vi "Update.vi"() -> ()   [LabVIEW 2015]
uses:
  <vilib>/zip/NI_Unzip.lvlib
panel:
  out "String":string
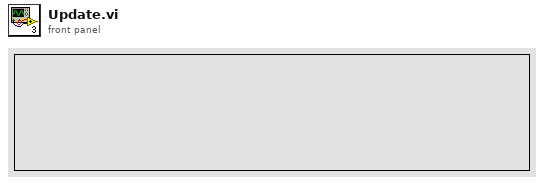
[diagram p1: front panel]
types:
  T1 = enum16{"open", "replace", "create", "open or create", "replace or create", "replace or create with confirmation"}
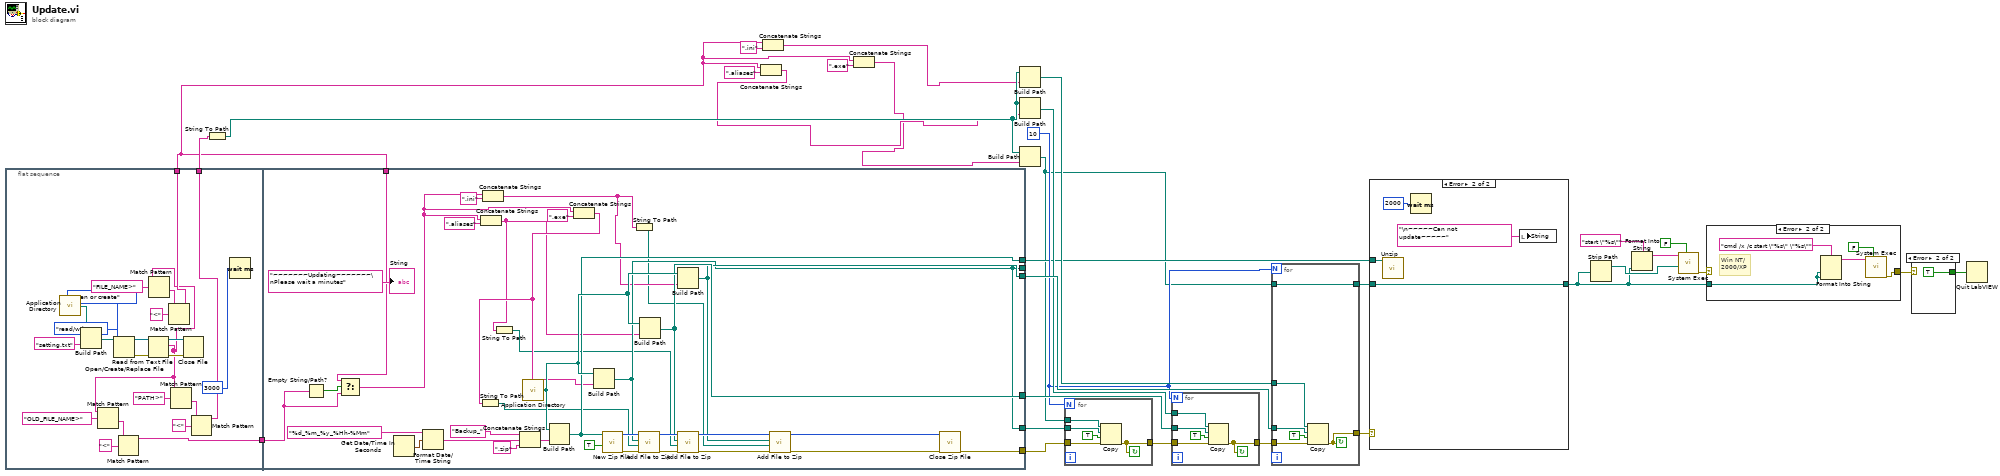
[diagram p0: block diagram]
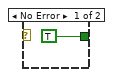
[diagram p2: hidden frame]
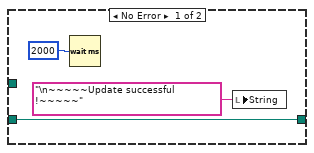
[diagram p4: hidden frame]
diagram:
  w23 = 10
  n1 = flat-sequence {
    tunnel: [w41] -> w7
    tunnel: [w37] -> w2
    tunnel: [w32] -> w3
    tunnel: [w68] -> w31
    tunnel: [w74] -> w30
    tunnel: [w73] -> w29
    tunnel: [w71] -> w28
    tunnel: [w70] -> w22
    tunnel: [w68] -> _
    tunnel: w3 -> [w65]
    tunnel: w2 -> [w66]
    frame #0 {
      n2 = call <vilib>:"Application Directory.vi"() -> ("Application Directory"=w53:path)
      n3 = Build Path(base path=w53, name or relative path="setting.txt") -> (appended path=w51:path)
      n4 = Open/Create/Replace File(file path (use dialog)=w51, operation (0:open)=T1."open or create", access (0:read/write)=enum16{"read/write", "read-only", "write-only"}."read/write") -> (refnum out=w48:refnum<file>, error out=w47:errorcluster)  [unwired: 3 in, 1 out]
      n5 = Read from Text File(file (use dialog)=w48, error in=w47) -> (refnum out=w46:refnum<file>, text=w33:string, error out=w45:errorcluster)  [unwired: 2 in, 1 out]
      n6 = Match Pattern(string=w33, regular expression="OLD_FILE_NAME>") -> (after substring=w35:string)  [unwired: 1 in, 3 out]
      n7 = Match Pattern(string=w35, regular expression="<") -> (before substring=w32:string)  [unwired: 1 in, 3 out]
      n8 = Match Pattern(string=w33, regular expression="FILE_NAME>") -> (after substring=w39:string)  [unwired: 1 in, 3 out]
      n9 = Match Pattern(string=w39, regular expression="<") -> (before substring=w37:string)  [unwired: 1 in, 3 out]
      n10 = Match Pattern(string=w33, regular expression="PATH>") -> (after substring=w43:string)  [unwired: 1 in, 3 out]
      n11 = Close File(refnum=w46, error in=w45) -> ()  [unwired: 2 out]
      n12 = Match Pattern(string=w43, regular expression="<") -> (before substring=w41:string)  [unwired: 1 in, 3 out]
      n13 = Wait (ms)(milliseconds to wait=u32 3000) -> ()  [unwired: 1 out]
    }
    frame #1 {
      n14 = Empty String/Path?(string/path=w65) -> (empty?=w67:bool)
      n15 = Select(t=w66, s=w67, f=w65) -> (s? t:f=w61:string)
      n16 = Get Date/Time In Seconds() -> (seconds since 1Jan1904=w89:timestamp)
      n17 = Format Date/Time String(time format string (%c)="%d_%m_%y_%Hh-%Mm", seconds (now)=w89) -> (date/time string=w87:string)  [unwired: 1 in]
      n18 = Concatenate Strings(w61, ".aliases" ("string")) -> (w57:string)
      n19 = Concatenate Strings(w61, ".ini" ("string")) -> (w56:string)
      n20 = String To Path(string=w57) -> (path=w58:path)
      n21 = Concatenate Strings("Backup_" ("string"), w87, ".zip" ("string")) -> (w72:string)
      n22 = call <vilib>:"Application Directory.vi"() -> ("Application Directory"=w86:path)
      n23 = Build Path(base path=w86, name or relative path=w72) -> (appended path=w70:path)
      n24 = Concatenate Strings(w61, ".exe" ("string")) -> (w60:string)
      n25 = String To Path(string=w60) -> (path=w59:path)
      n26 = Build Path(base path=w86, name or relative path=w60) -> (appended path=w68:path)
      n27 = call <vilib>:"New Zip File.vi"("confirm overwrite? (F)"=TRUE, "target"=w70) -> ("error out"=w81:errorcluster, "zip file out"=w84:i64)  [unwired: 3 in, 1 out]
      n28 = String To Path(string=w56) -> (path=w55:path)
      n29 = call <vilib>:"Add File to Zip.vi"("error in (no error)"=w81, "destination path in zip"=w59, "source file path"=w68, "zip file in"=w84) -> ("error out"=w80:errorcluster, "zip file out"=w83:i64)  [unwired: 6 in]
      n30 = Build Path(base path=w86, name or relative path=w57) -> (appended path=w74:path)
      n31 = Build Path(base path=w86, name or relative path=w56) -> (appended path=w73:path)
      n32 = call <vilib>:"Add File to Zip.vi"("error in (no error)"=w80, "destination path in zip"=w58, "source file path"=w74, "zip file in"=w83) -> ("error out"=w79:errorcluster, "zip file out"=w82:i64)  [unwired: 6 in]
      n33 = call <vilib>:"Add File to Zip.vi"("error in (no error)"=w79, "destination path in zip"=w55, "source file path"=w73, "zip file in"=w82) -> ("error out"=w77:errorcluster, "zip file out"=w78:i64)  [unwired: 6 in]
      n34 = call <vilib>:"Close Zip File.vi"("error in (no error)"=w77, "zip file in"=w78) -> ("error out"=w71:errorcluster)  [unwired: 5 in]
      "String" <- "~~~~~~~Updating~~~~~~~\nPlease wait a minutes" ("String")
    }
  }
  n35 = String To Path(string=w7) -> (path=w8:path)
  n36 = Concatenate Strings(w2, ".aliases" ("string")) -> (w5:string)
  n37 = Concatenate Strings(w2, ".ini" ("string")) -> (w6:string)
  n38 = Concatenate Strings(w2, ".exe" ("string")) -> (w4:string)
  n39 = Build Path(base path=w8, name or relative path=w6) -> (appended path=w26:path)
  n40 = Build Path(base path=w8, name or relative path=w5) -> (appended path=w27:path)
  n41 = Build Path(base path=w8, name or relative path=w4) -> (appended path=w1:path)
  n42 = for {
    N: w23 -> [_]
    tunnel: w1 -> [w94]
    tunnel: w31 -> [w93]
    tunnel: w28 -> [w91]
    tunnel: [w90] -> w25
    stop <- w90 continue-if-true
    n43 = Copy(8:w91, 9:TRUE ("overwrite (F)"), 10:w93, 11:w94) -> (0:w90:errorcluster)  [unwired: 1 in, 2 out]
  }
  n44 = for {
    N: w23 -> [_]
    tunnel: w27 -> [w99]
    tunnel: w30 -> [w98]
    tunnel: w25 -> [w96]
    tunnel: [w95] -> w24
    stop <- w95 continue-if-true
    n45 = Copy(8:w96, 9:TRUE ("overwrite (F)"), 10:w98, 11:w99) -> (0:w95:errorcluster)  [unwired: 1 in, 2 out]
  }
  n46 = for {
    N: w23 -> [_]
    tunnel: w26 -> [w105]
    tunnel: w29 -> [w104]
    tunnel: w24 -> [w102]
    tunnel: [w101] -> w21
    tunnel: [w100] -> w13
    tunnel: w1 -> [w100]
    stop <- w101 continue-if-true
    n47 = Copy(8:w102, 9:TRUE ("overwrite (F)"), 10:w104, 11:w105) -> (0:w101:errorcluster)  [unwired: 1 in, 2 out]
  }
  n48 = case shown="Error" w21 {
    tunnel: w22 -> [_ w112]
    tunnel: [w106 w109] -> w14
    tunnel: w13 -> [w106 w109]
    frame No Error {
      n49 = Wait (ms)(milliseconds to wait=u32 2000) -> ()  [unwired: 1 out]
      n50 = local write "String"("\n~~~~~Update successful !~~~~~" ("message")) -> ()
    }
    frame Error {
      n51 = call <vilib>:"Unzip.vi"("Zip file"=w112) -> ()  [unwired: 8 in, 3 out]
      n52 = Wait (ms)(milliseconds to wait=u32 2000) -> ()  [unwired: 1 out]
      n53 = local write "String"("\n~~~~~Can not update~~~~~" ("message")) -> ()
    }
  }
  n54 = Strip Path(path=w14) -> (stripped path=w18:path)  [unwired: 1 out]
  n55 = Format Into String(format string="start \"%s\"", w14) -> (resulting string=w17:string)  [unwired: 2 in, 1 out]
  n56 = call <vilib>:"System Exec.vi"("wait until completion? (T)"=FALSE ("Wait until done"), "working directory"=w18, "command line"=w17) -> ("error out"=w19:errorcluster)  [unwired: 5 in, 3 out]
  n57 = case shown="Error" w19 {
    selector: w19 -> [w113 _]
    tunnel: w14 -> [_ w115]
    tunnel: [w113 w114] -> w20
    frame No Error {
    }
    frame Error {
      # "Win NT/\n2000/XP"
      n58 = Format Into String(format string="cmd /x /c start \"%s\" \"%s\"", w115, w115) -> (resulting string=w116:string)  [unwired: 2 in, 1 out]
      n59 = call <vilib>:"System Exec.vi"("wait until completion? (T)"=FALSE ("Wait until done"), "command line"=w116) -> ("error out"=w114:errorcluster)  [unwired: 6 in, 3 out]
    }
  }
  n60 = case shown="Error" w20 {
    tunnel: [TRUE TRUE] -> w12
    frame No Error {
    }
    frame Error {
    }
  }
  n61 = Quit LabVIEW(quit? (T)=w12) -> ()
